vi "Delete UI Reference Mal.vi"(8 "error in (no error)":errorcluster, 10 "Panel":string, 11 "UI Reference Wrapper in":refnum<class "UI Reference Wrapper.lvclass">) -> (0 "error out":errorcluster, 1 "Index":i32, 2 "deleted portion":cluster{"VI Refnum":refnum<vi>, "Name":string}, 3 "UI Reference Wrapper out":refnum<class "UI Reference Wrapper.lvclass">)   [LabVIEW 2019, in "UI Reference Wrapper.lvclass"]
uses:
  UI Reference Wrapper.lvclass
  UI Reference Wrapper.lvclass/UI Reference Wrapper.ctl
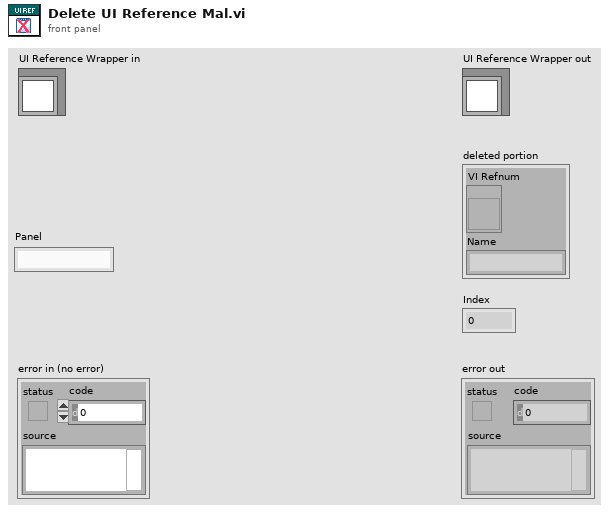
[diagram p1: front panel]
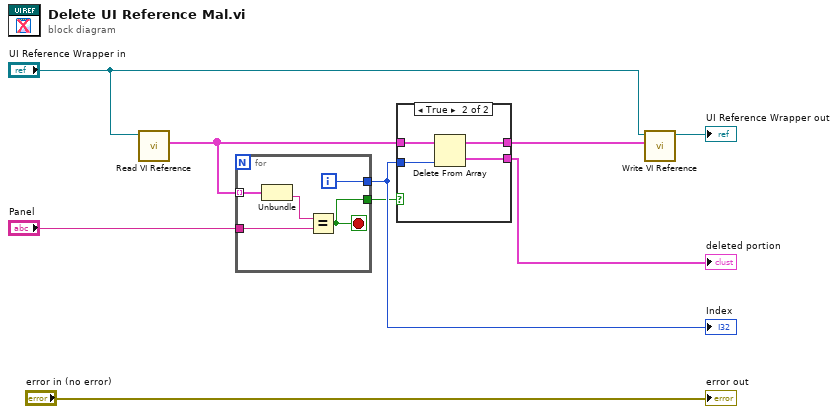
[diagram p0: block diagram]
diagram:
  n1 = call "Read VI Reference.vi"("UI Reference Wrapper in"="UI Reference Wrapper in") -> ("VI Reference Wrappers"=w9:cluster{"VI Refnum":refnum<vi>, "Name":string}[])  [unwired: 8 in, 2 out]
  n2 = for {
    tunnel: w9 -> [w14] mode=indexing
    tunnel: "Panel" -> [w13]
    tunnel: [w12] -> w3
    tunnel: [w11] -> w2
    i -> [w12]
    stop <- w11 stop-if-true
    n3 = Unbundle(w14) -> ("Name"=w10:string)  [unwired: 1 out]
    n4 = Equal?(x=w10, y=w13) -> (x = y?=w11:bool)
  }
  "Index" <- w3
  n5 = case shown="True" w2 {
    tunnel: w9 -> [w15 w19]
    tunnel: [w15 w18] -> w8
    tunnel: [_ w17] -> w5
    tunnel: w3 -> [_ w16]
    frame False {
    }
    frame True {
      n6 = Delete From Array(array=w19, index=w16) -> (deleted portion=w17:cluster{"VI Refnum":refnum<vi>, "Name":string}, array with subset deleted=w18:cluster{"VI Refnum":refnum<vi>, "Name":string}[])  [unwired: 1 in]
    }
  }
  "deleted portion" <- w5
  n7 = call "Write VI Reference.vi"("VI Reference Wrappers"=w8, "UI Reference Wrapper in"="UI Reference Wrapper in") -> ("UI Reference Wrapper out"=→"UI Reference Wrapper out":refnum<class "UI Reference Wrapper.lvclass">)  [unwired: 8 in, 1 out]
  "error out" <- "error in (no error)"
